vi "TimeSampleDlgg.vi"() -> (2 "定时采样信息":T1)   [LabVIEW 2014, in "Sample.lvlib"]
uses:
  Sample.lvlib
  DataBase/DataBase.lvlib
panel:
  in  "备注":string
  out "电压范围":string
  in  "取消按钮":bool
  in  "确定按钮":bool
  in  "电源频率（Hz）":string="1"
  in  "电源电压":string
  in  "分钟":u16(ring) items=["0", "01", "02", "03", "04", "05", "06", "07", "08", "09", "10", "11", "12", "13", "14", "15", "16", "17", "18", "19", "20", "21", "22", "23", "24", "25", "26", "27", "28", "29", "30", "31", "32", "33", "34", "35", "36", "37", "38", "39", "40", "41", "42", "43", "44", "45", "46", "47", "48", "49", "50", "51", "52", "53", "54", "55", "56", "57", "58", "59"]
  in  "时":u16(ring) items=["1", "2", "3", "4", "5", "6", "7", "8", "9", "10", "11", "12", "13", "14", "15", "16", "17", "18", "19", "20", "21", "22", "23", "24"]
  in  "检测区域":string(combo)
  in  "是否启动":string(combo)="是"
  in  "检测位置":string(combo)="上层膜检测"
  in  "OK":bool
  # "检测时间"
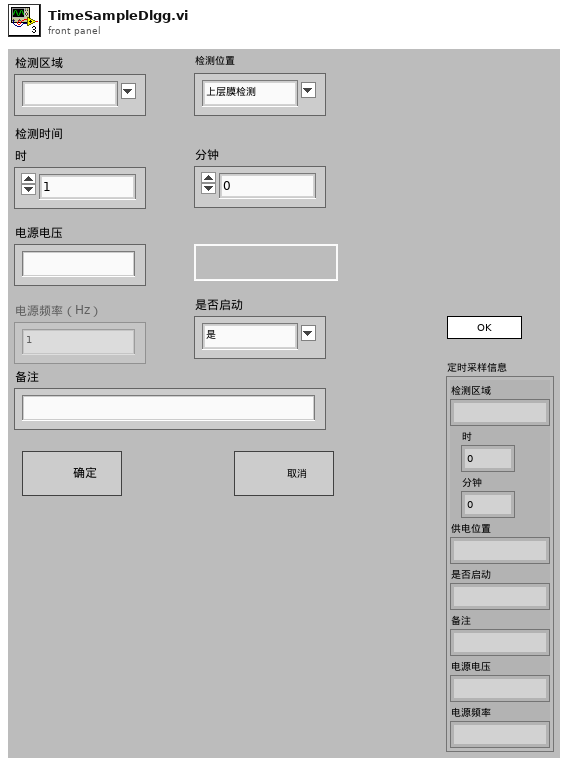
[diagram p1: front panel]
types:
  T1 = cluster{"检测区域":string, "时":u16, "分钟":u16, "供电位置":string, "是否启动":string, "备注":string, "电源电压":string, "电源频率":string}
  T2 = enum32{"invalid app kind", "Development System", "Run Time System", "Student Edition", "Embedded LabVIEW", "Evaluation", "Custom"}
  T3 = enum32{"Invalid", "Standard", "Closed", "Hidden", "Minimized", "Maximized"}
  T4 = cluster{"Core":cluster{"Current VI Reference":refnum<vi>, "Close Panel on Exit?":bool}, "Your Boolean data":bool, "Your string data":string, "AreaName":string, "SampleAreaName":string[], "定时采样信息":cluster{"检测区域":string, "时":u16, "分钟":u16, "供电位置":string, "是否启动":string, "备注":string, "电源电压":string, "电源频率":string}, "电源倍数":string, "最大电压值":i32}
  T5 = cluster{"Current VI Reference":refnum<vi>, "Close Panel on Exit?":bool}
  T6 = cluster{string, "检测区域":string, "供电位置":string, string, string, "是否启动":string, "电源电压":string, "电源频率":string, "备注":string}
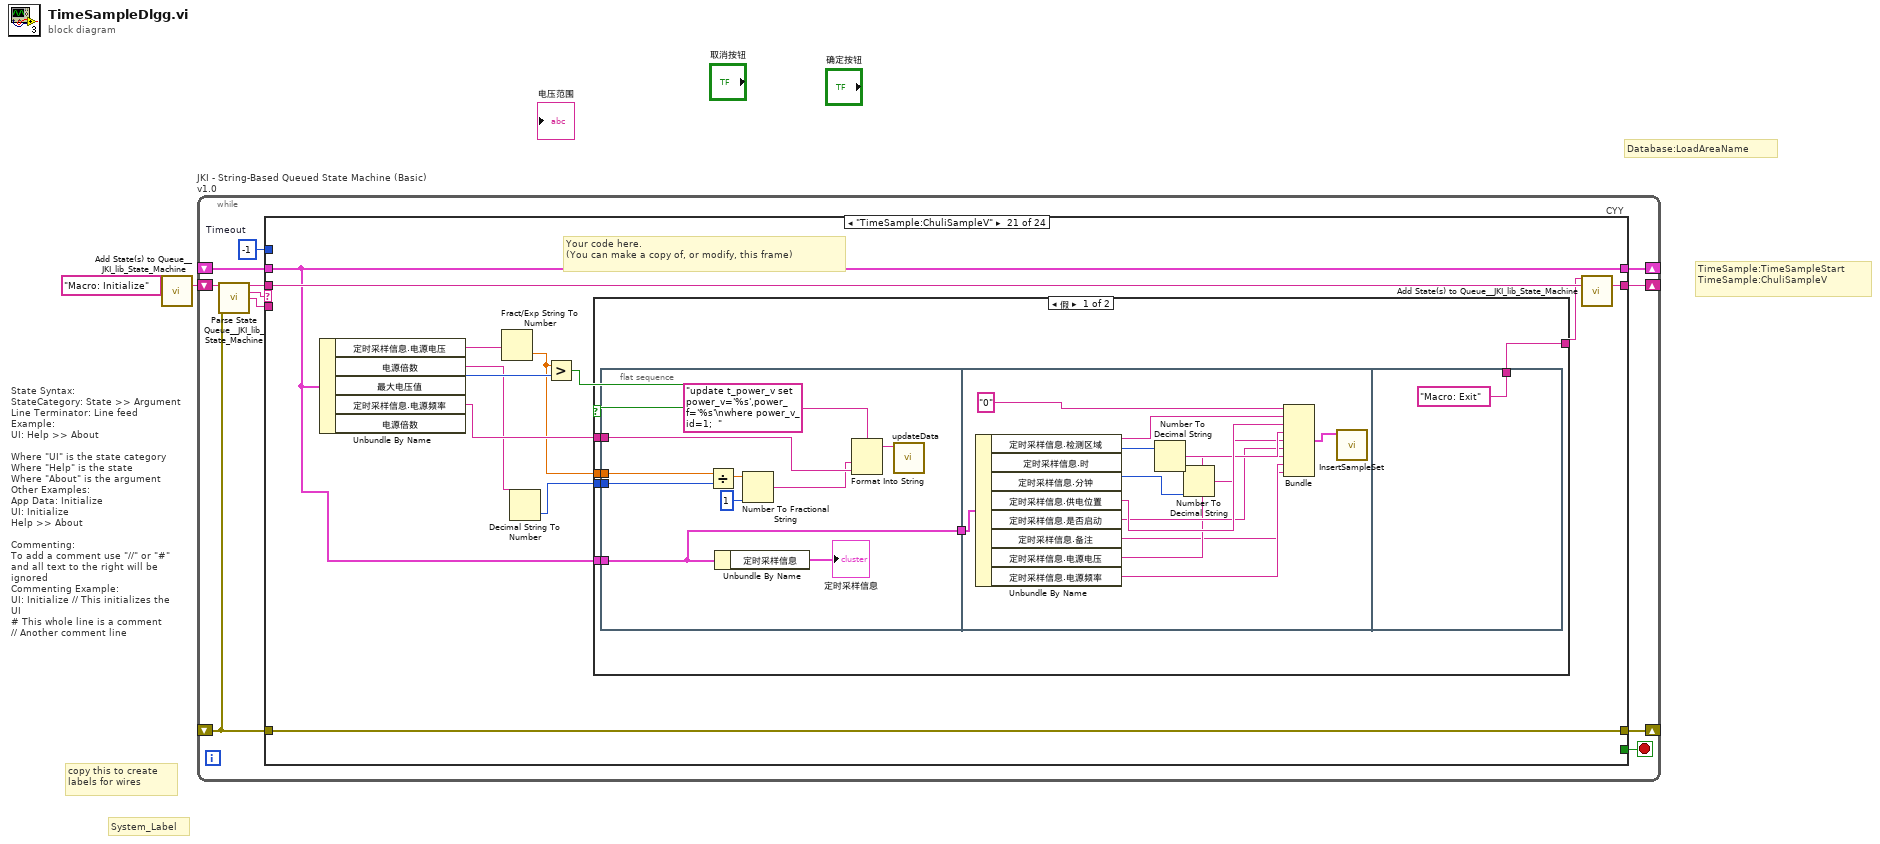
[diagram p0: block diagram]
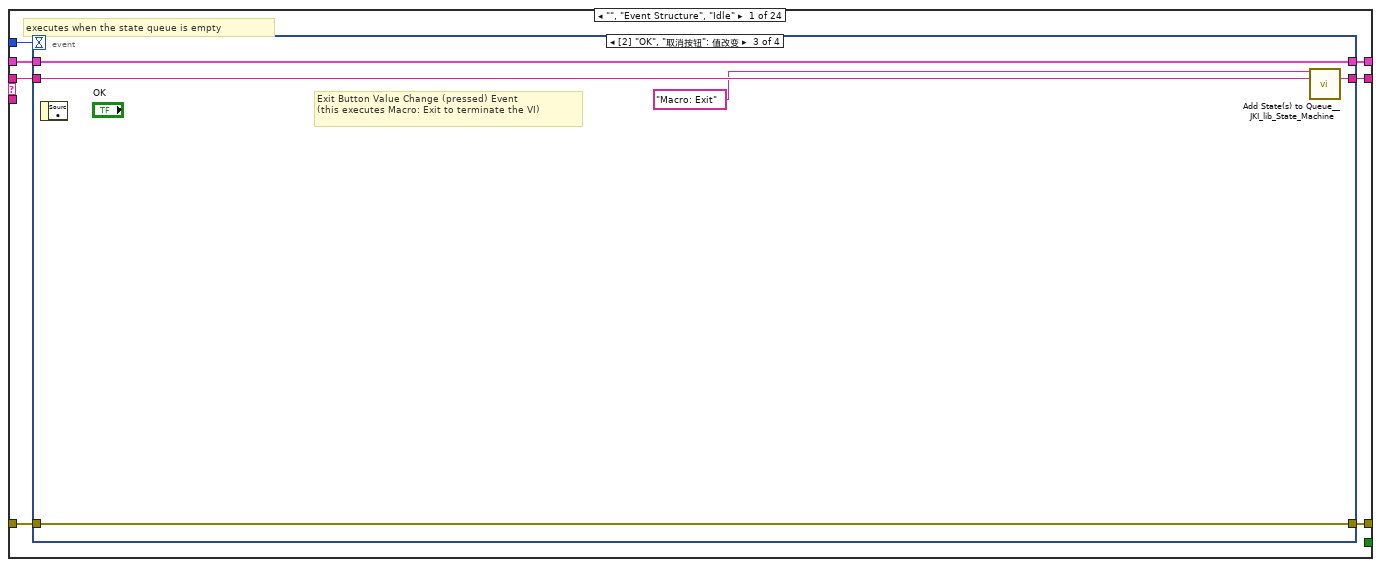
[diagram p2: hidden frame]
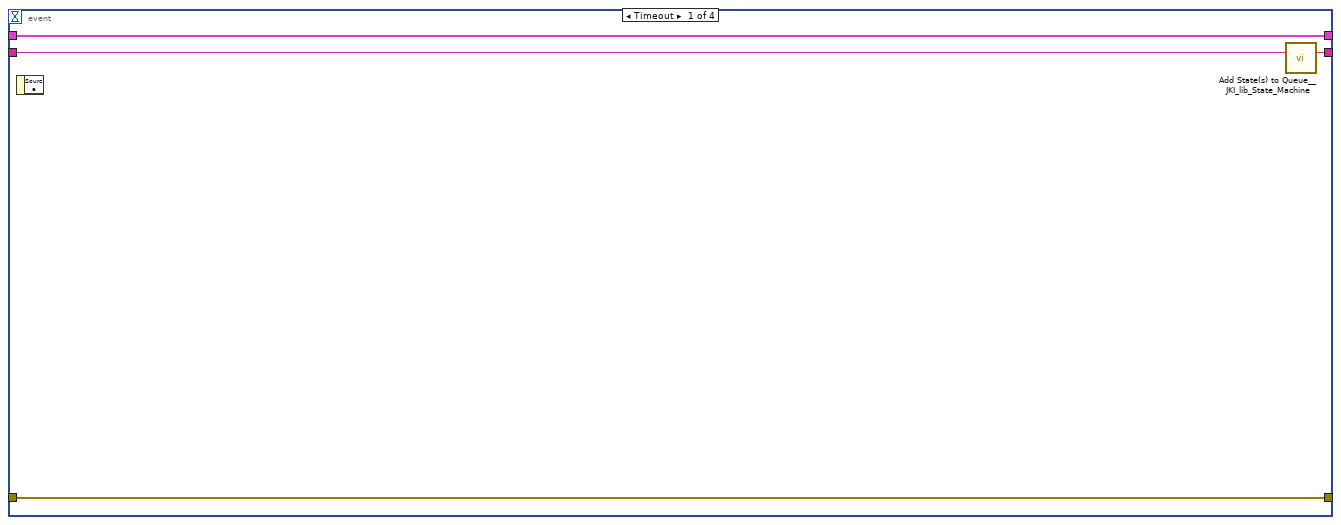
[diagram p3: hidden frame]
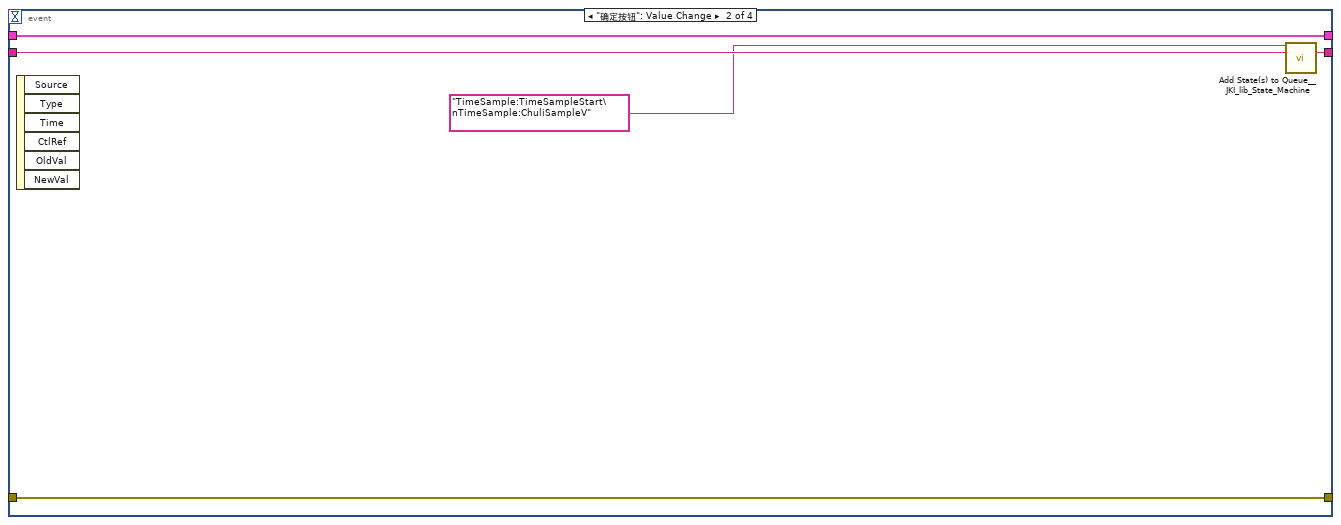
[diagram p4: hidden frame]
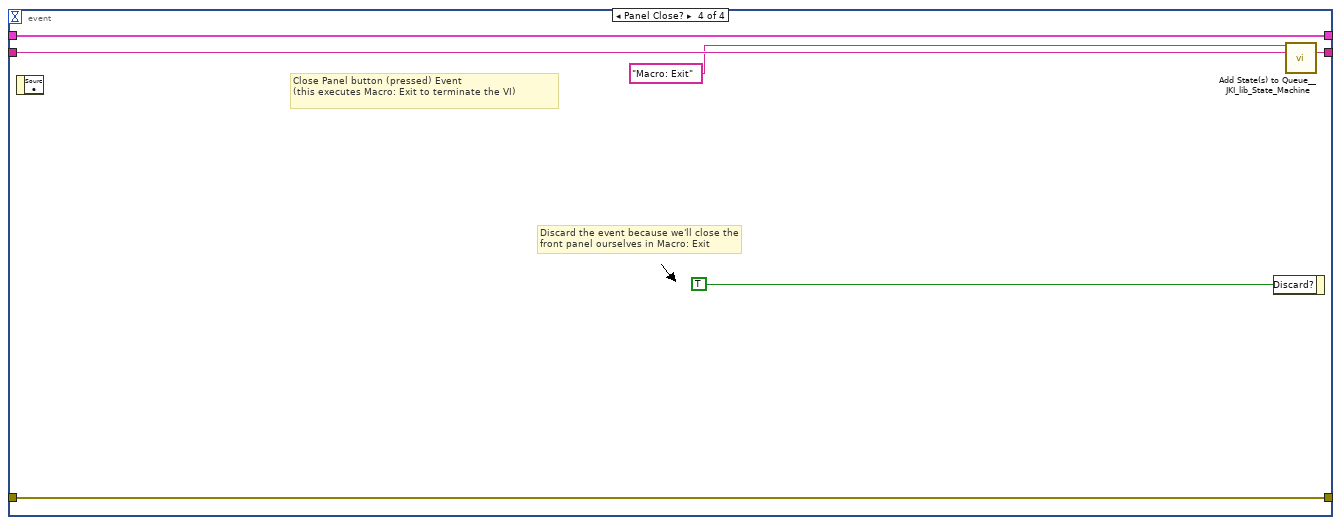
[diagram p5: hidden frame]
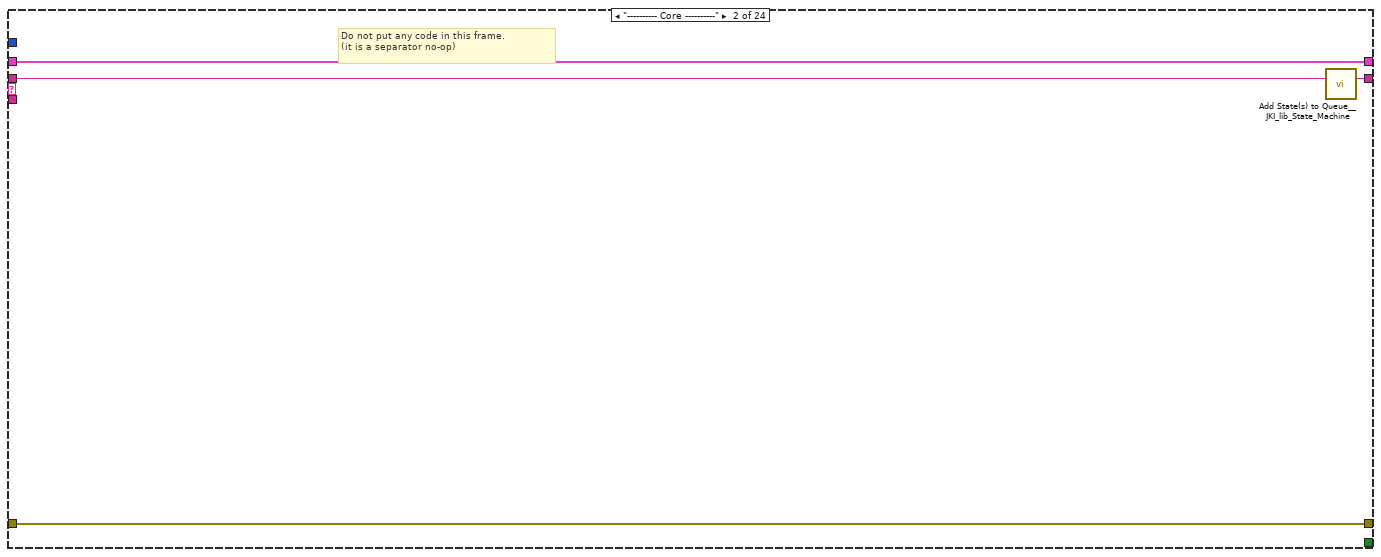
[diagram p6: hidden frame]
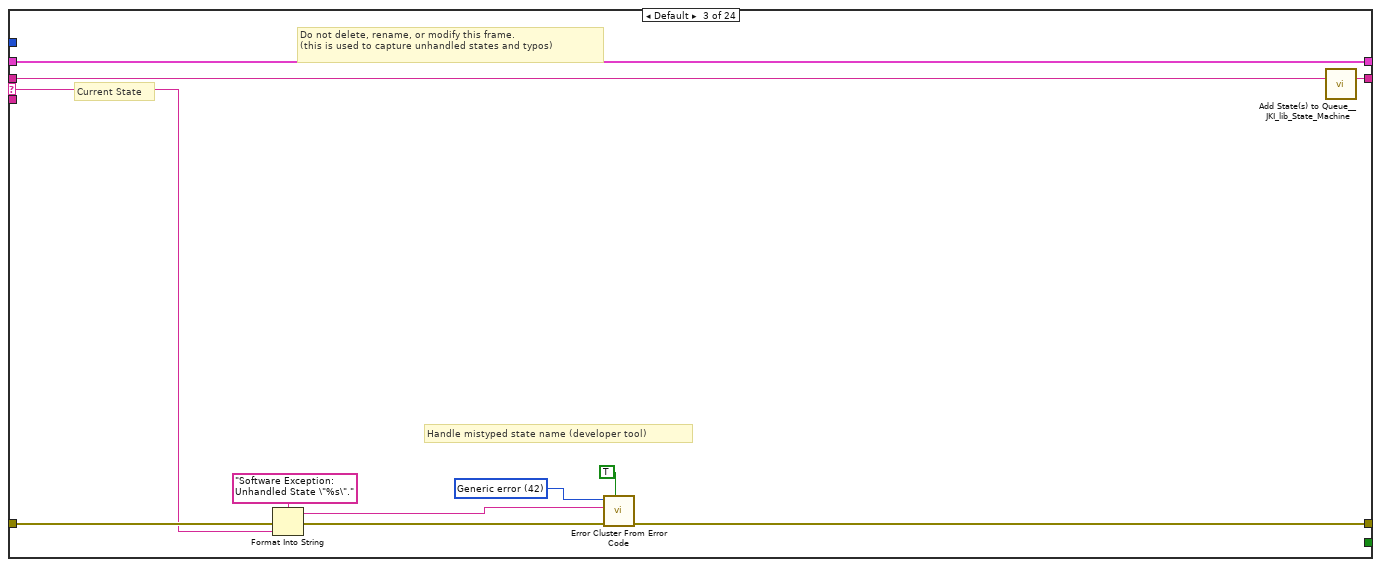
[diagram p7: hidden frame]
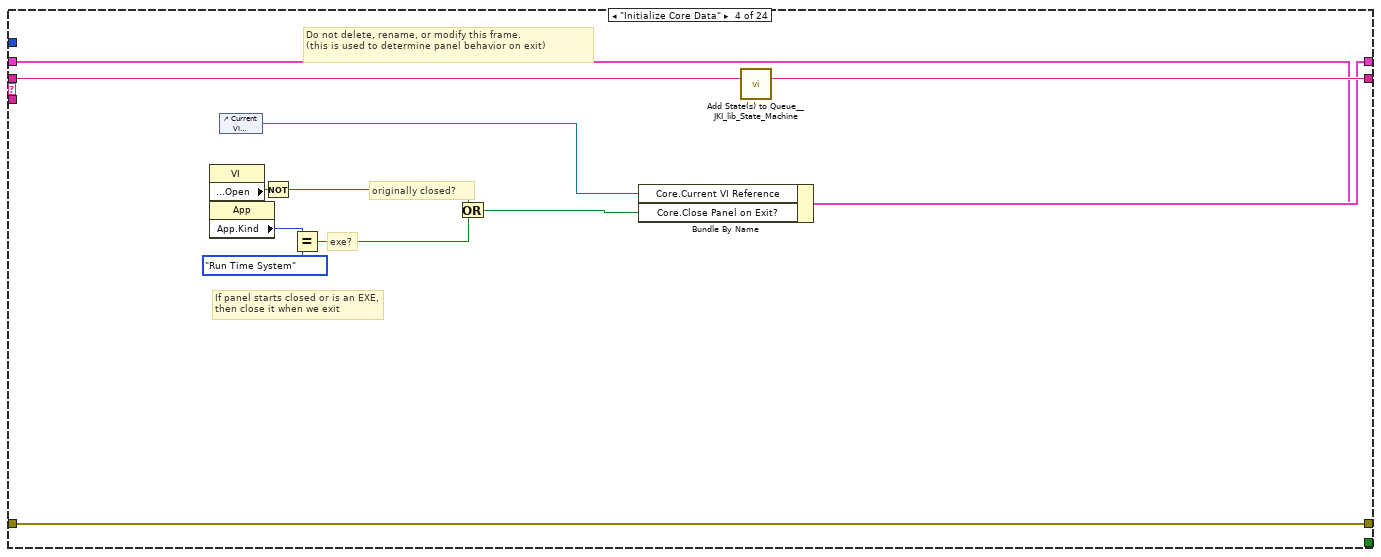
[diagram p8: hidden frame]
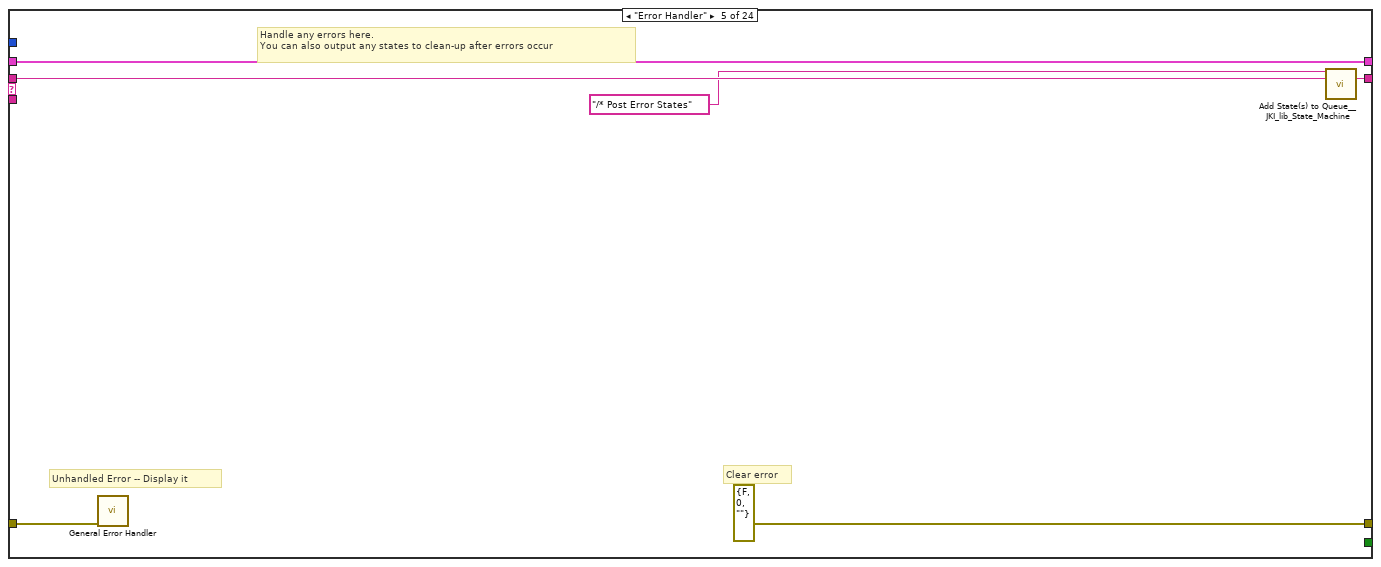
[diagram p9: hidden frame]
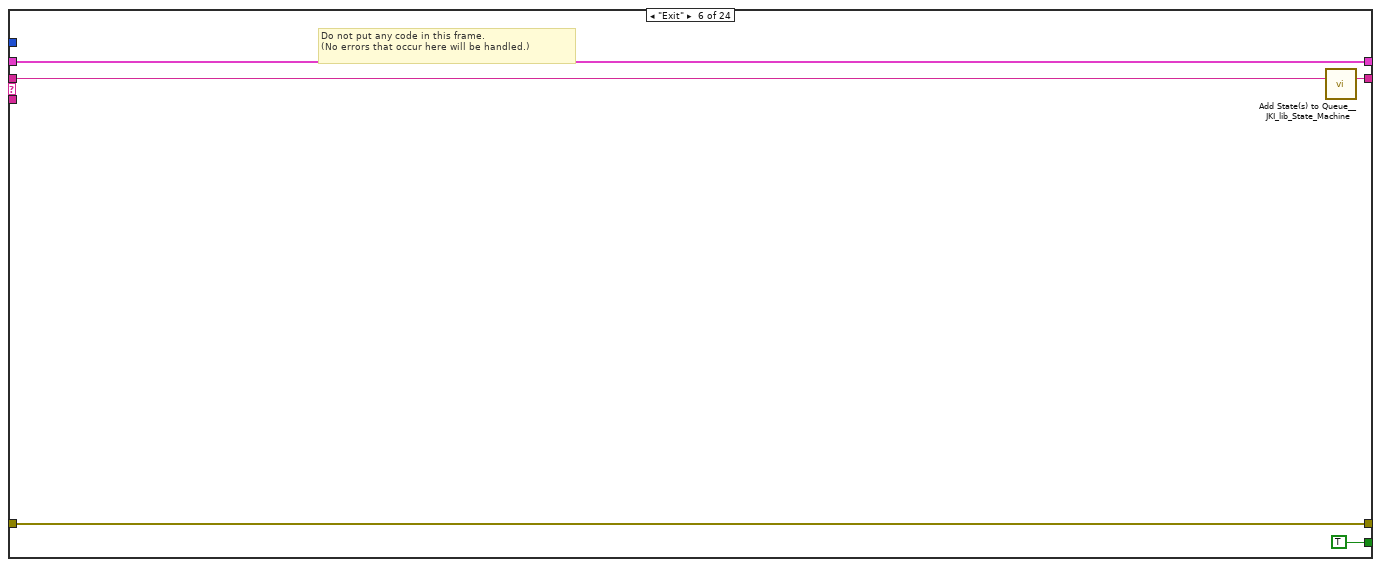
[diagram p10: hidden frame]
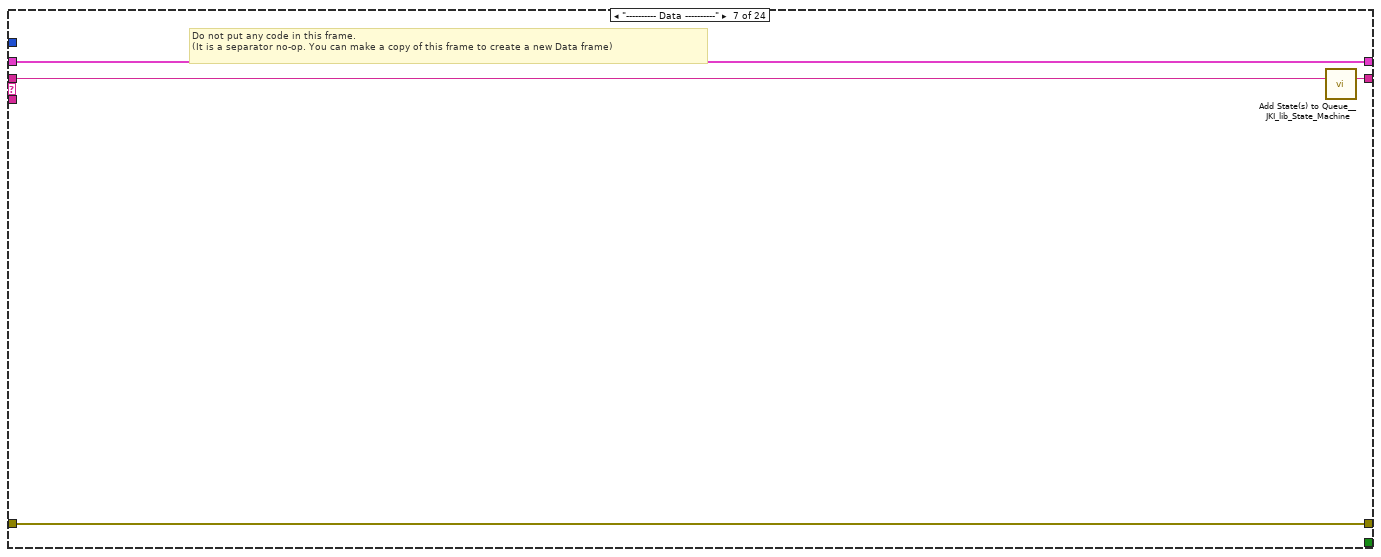
[diagram p11: hidden frame]
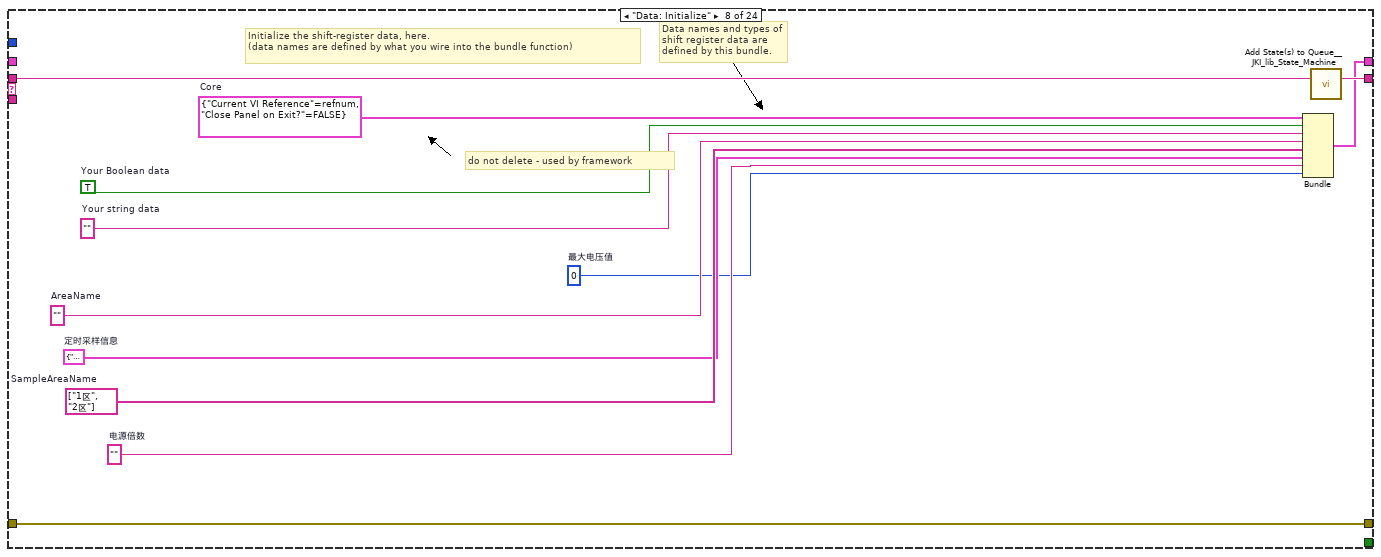
[diagram p12: hidden frame]
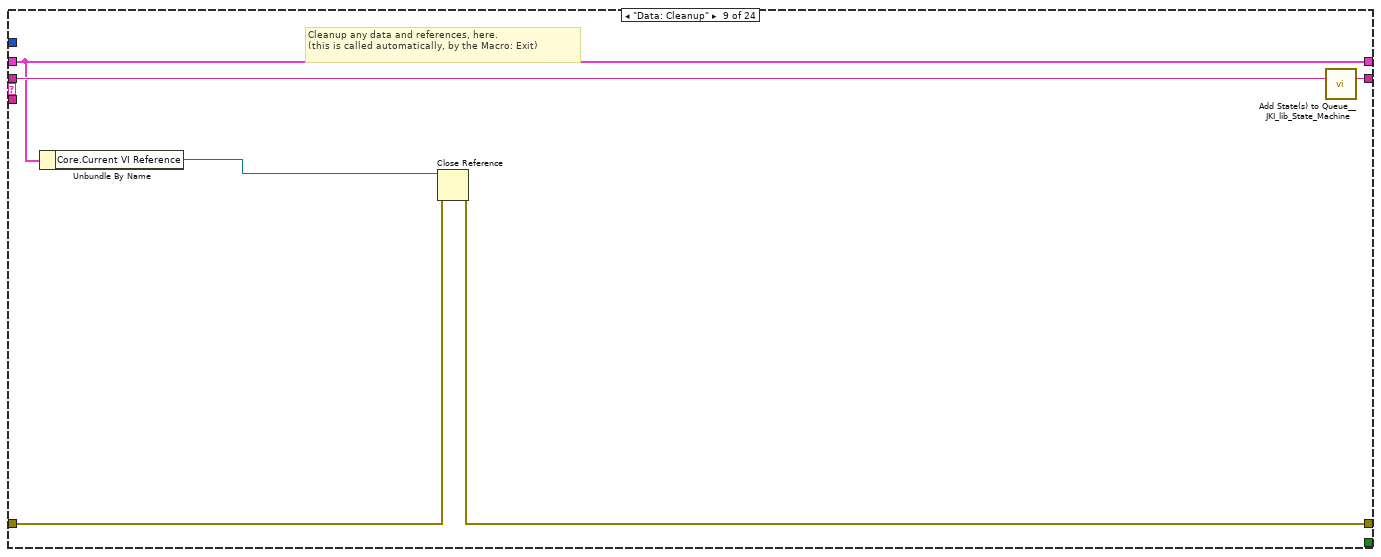
[diagram p13: hidden frame]
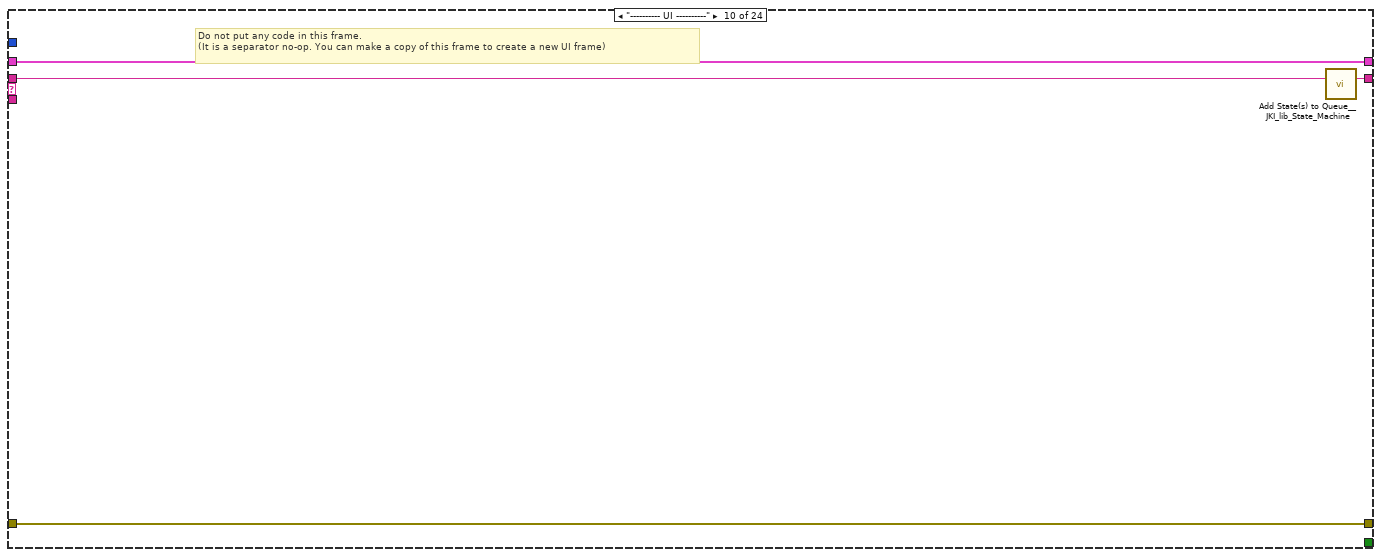
[diagram p14: hidden frame]
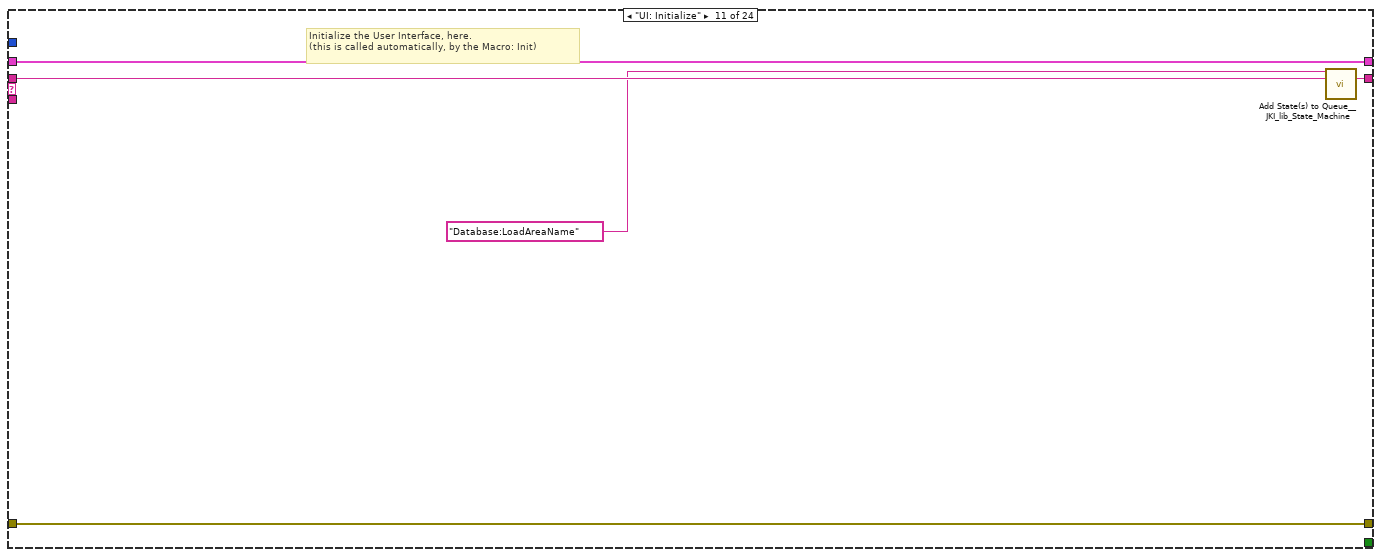
[diagram p15: hidden frame]
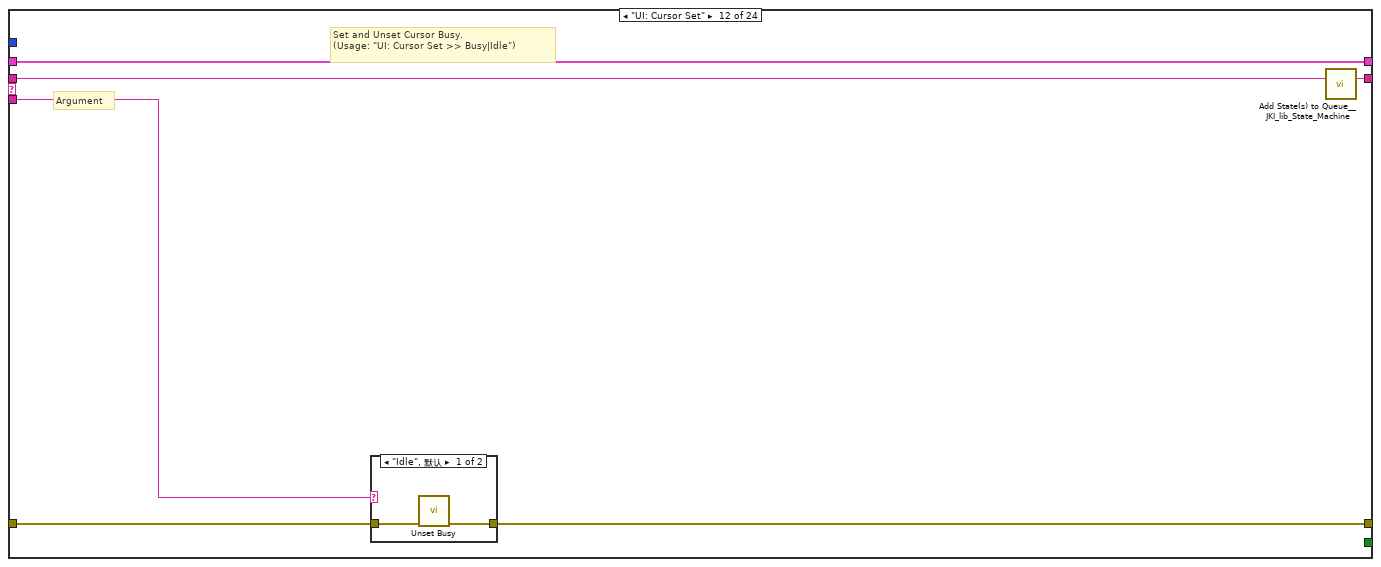
[diagram p16: hidden frame]
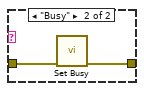
[diagram p17: hidden frame]
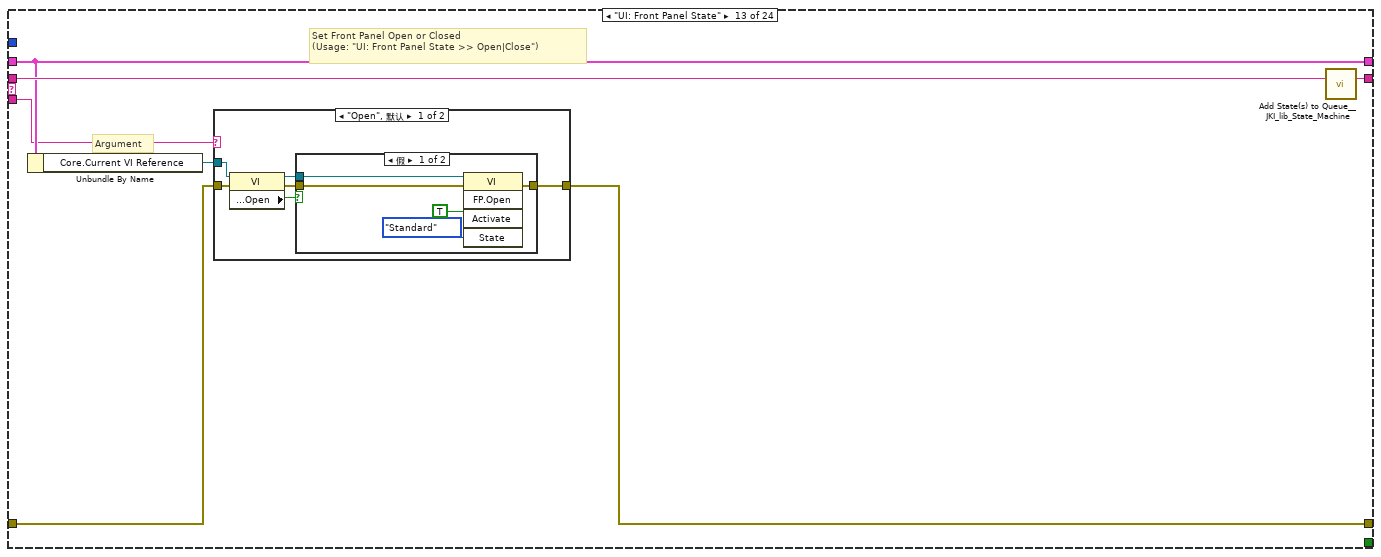
[diagram p18: hidden frame]
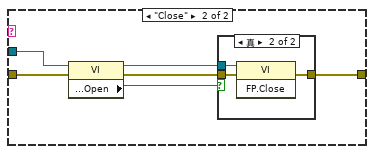
[diagram p20: hidden frame]
diagram:
  # "TimeSample:TimeSampleStart\nTimeSample:ChuliSampleV"
  # "Database:LoadAreaName"
  # "State Syntax:\nStateCategory: State >> Argument\nLine Terminator: Line feed\nExample:\nUI: Help >> About\n\nWhere \"UI\" is the state category\nWhere \"Help\" is the state\nWhere \"About\" is the argument\nOther Examples:\nApp Data: Initialize\nUI: Initialize\nHelp >> About\n\nCommenting:\nTo add a comment use \"//\" or \"#\" and all text to the right will be ignored\nCommenting Example:\nUI: Initialize // This initializes the UI\n# This whole line is a comment\n// Another comment line"
  # "copy this to create labels for wires"
  # "System_Label"
  n1 = call <vilib>:"Add State(s) to Queue__JKI_lib_State_Machine.vi"("State(s) in (\"\")"="Macro: Initialize") -> ("States Out"=w2:string)  [unwired: 14 in]
  n2 = while "JKI - String-Based Queued State Machine (Basic) v1.0" {
    shift-right: [w6] -> _
    shift-left: _ -> [w5]
    shift-right: [w9] -> _
    shift-left: _ -> [w3]
    shift-right: [w8] -> _
    shift-left: w2 -> [w10]
    stop <- w7 stop-if-true
    w4 = -1  # Timeout
    # "CYY"
    n3 = call <vilib>:"Parse State Queue__JKI_lib_State_Machine.vi"("State Queue"=w10, "Error In (no error)"=w3) -> ("Remaining States"=w12:string, "Current State"=w13:string, "Arguments"=w11:string)  [unwired: 11 in]
    n4 = case shown="\"TimeSample:ChuliSampleV\"" w13 {
      selector: w13 -> [_ _ w45 _ _ _ _ _ _ _ _ _ _ _ _ _ _ _ _ _ _ _ _ _]
      tunnel: w12 -> [w20 w44 w49 w67 w73 w78 w82 w94 w100 w104 w109 w115 w126 w152 w157 w167 w171 w175 w179 w183 w195 w241 w245 w255]
      tunnel: w11 -> [_ _ _ _ _ _ _ _ _ _ _ w110 w120 _ _ _ _ _ _ _ _ _ _ _]
      tunnel: w5 -> [w18 w41 w47 w58 w70 w76 w79 _ w95 w101 w107 w113 w122 w149 w154 w164 w168 w172 w176 w180 w184 w229 w242 w252]
      tunnel: [w17 w42 w51 w64 errorcluster {"status"=FALSE, "code"=0, "source"=""} ("error out") w75 w80 w91 w96 w102 w106 w111 w123 w150 w155 w165 w169 w173 w177 w181 w193 w239 w243 w253] -> w9
      tunnel: w3 -> [w16 w42 w50 w64 w69 w75 w80 w91 w97 w102 w106 w112 w124 w150 w155 w165 w169 w173 w177 w181 w193 w239 w243 w253]
      tunnel: [w19 w43 w48 w66 w72 w77 w81 w93 w99 w103 w108 w114 w125 w151 w156 w166 w170 w174 w178 w182 w194 w240 w244 w254] -> w8
      tunnel: [_ _ _ _ _ TRUE _ _ _ _ _ _ _ _ _ _ _ _ _ _ _ _ _ _] -> w7
      tunnel: [w15 w41 w47 w65 w70 w76 w79 w92 w95 w101 w107 w113 w122 w149 w154 w164 w168 w172 w176 w180 w184 w238 w242 w251] -> w6
      tunnel: w4 -> [w14 _ _ _ _ _ _ _ _ _ _ _ _ _ _ _ _ _ _ _ _ _ _ _]
      frame "", "Event Structure", "Idle" {
        # "executes when the state queue is empty"
        n5 = event shown="[2] \"OK\", \"取消按钮\": 值改变" {
          selector: _ -> [_ _ _ _]
          dyn-events: _ -> [_ _ _ _]
          timeout: w14 -> [_ _ _ _]
          tunnel: w20 -> [w24 w29 w34 w40]
          tunnel: [w23 w28 w33 w39] -> w19
          tunnel: w18 -> [w21 w26 w31 w37]
          tunnel: [w22 w27 w32 w38] -> w17
          tunnel: w16 -> [w22 w27 w32 w38]
          tunnel: [w21 w26 w31 w37] -> w15
          event Timeout {
            n6 = event-data() -> ()  [unwired: 1 in, 1 out]
            n7 = call <vilib>:"Add State(s) to Queue__JKI_lib_State_Machine.vi"("State(s) in (\"\")"=w24) -> ("States Out"=w23:string)  [unwired: 14 in]
          }
          event "确定按钮": Value Change {
            n8 = event-data() -> ()  [unwired: 1 in, 6 out]
            n9 = call <vilib>:"Add State(s) to Queue__JKI_lib_State_Machine.vi"("State(s) in Front (\"\")"="TimeSample:TimeSampleStart\nTimeSample:ChuliSampleV", "State(s) in (\"\")"=w29) -> ("States Out"=w28:string)  [unwired: 13 in]
          }
          event "OK", "取消按钮": Value Change {
            # "Exit Button Value Change (pressed) Event\n(this executes Macro: Exit to terminate the VI)"
            n10 = event-data() -> ()  [unwired: 1 in, 1 out]
            n11 = call <vilib>:"Add State(s) to Queue__JKI_lib_State_Machine.vi"("State(s) in Front (\"\")"="Macro: Exit", "State(s) in (\"\")"=w34) -> ("States Out"=w33:string)  [unwired: 13 in]
          }
          event Panel Close? {
            # "Discard the event because we'll close the front panel ourselves in Macro: Exit"
            # "Close Panel button (pressed) Event\n(this executes Macro: Exit to terminate the VI)"
            n12 = event-data() -> ()  [unwired: 1 in, 1 out]
            n13 = event-data("Discard?"=TRUE) -> ()  [unwired: 1 in, 1 out]
            n14 = call <vilib>:"Add State(s) to Queue__JKI_lib_State_Machine.vi"("State(s) in Front (\"\")"="Macro: Exit", "State(s) in (\"\")"=w40) -> ("States Out"=w39:string)  [unwired: 13 in]
          }
        }
      }
      frame "---------- Core ----------" {
        # "Do not put any code in this frame.\n(it is a separator no-op)"
        n15 = call <vilib>:"Add State(s) to Queue__JKI_lib_State_Machine.vi"("State(s) in (\"\")"=w44) -> ("States Out"=w43:string)  [unwired: 14 in]
      }
      frame Default {
        w54 = 42 items=["No error", "Argument error", "Memory is full", "Out of zone", "End of file", "File already open", "Generic file I/O error", "File not found", "File permission error", "Disk is full", "Duplicate path", "Too many files open", "System feature not enabled", "Resource file not found", "Cannot add resource", "Resource not found", "Image not found", "Image memory error", "Pen does not exist", "Config type invalid", "Config token not found", "Config parse error", "Config memory error", "Bad external code format", "Bad external code offset", "External code not present", "Null window", "Destroy window error", "Null menu", "Print aborted", "Bad print record", "Print driver error", "Windows error during printing", "Memory error during printing", "Print dialog error", "Generic print error", "Invalid device refnum", "Device not found", "Device parameter error", "Device unit error", "Cannot open device", "Device call aborted", "Generic error", "Cancelled by user", "Object ID too low", "Object ID too high", "Object not in heap", "Unknown heap", "Unknown object (invalid DefProc)", "Unknown object (DefProc not in table)", "Message out of range", "Invalid (null) method", "Unknown message", "Manager call not supported", "Bad address", "Network operation in progress", "Network operation timed out", "Connection is busy", "Network attribute not supported", "Network error", "Address in use", "System out of memory", "Connection aborted", "Connection refused", "Not connected", "Already connected", "Connection closed", "Initialization error (interapplication manager)", "Bad occurrence", "Wait on unbound occurrence handler", "Occurrence queue overflow", "Datalog type conflict", "Unused", "Unrecognized type (interapplication manager)", "Memory corrupt", "Failed to make temporary DLL", "Old CIN version", "Drag socket not found", "Failed to load drop-object", "Failed to register OLE object", "Failed to release OLE object", "Format specifier type mismatch", "Unknown format specifier", "Too few format specifiers", "Too many format specifiers", "Scan failed", "Newer CIN version", "Error converting to variant", "Runtime menu error", "Password tampered", "Variant attribute not found", "Incompatible variant data type", "Event data is not available", "Event Store is not present", "Occurrence is not found", "Event Queue is not created", "Event info is not available", "Refnum passed is NULL", "Error retrieving Class GUID", "Error retrieving CoClass GUID", "Error retrieving TypeLib GUID.", "Bad built application magic bytes.", "Specific driver is different from the specific driver associated with the Logical Name.", "There is no session opened to the class driver.", "Max Error", "MAX - Error with config objects", "MAX - Error loading configuration", "MAX - Group not supported"]
        # "Current State"
        # "Do not delete, rename, or modify this frame.\n(this is used to capture unhandled states and typos)"
        # "Handle mistyped state name (developer tool)"
        n16 = Format Into String(format string="Software Exception: Unhandled State \"%s\"." ("message"), error in=w50, w45) -> (resulting string=w53:string, error out=w52:errorcluster)  [unwired: 1 in]
        n17 = call <vilib>:"Error Cluster From Error Code.vi"("show call chain? (False)"=TRUE, "error in (no error)"=w52, "error message (\"\")"=w53, "error code (0)"=w54) -> ("error out"=w51:errorcluster)  [unwired: 5 in]
        n18 = call <vilib>:"Add State(s) to Queue__JKI_lib_State_Machine.vi"("State(s) in (\"\")"=w49) -> ("States Out"=w48:string)  [unwired: 14 in]
      }
      frame "Initialize Core Data" {
        # "Do not delete, rename, or modify this frame.\n(this is used to determine panel behavior on exit)"
        # "originally closed?"
        # "exe?"
        # "If panel starts closed or is an EXE, then close it when we exit"
        n19 = property class="VI"() -> ("Front Panel.Open"=w63:bool)  [unwired: 2 in, 2 out]
        n20 = property class="App"() -> ("App.Kind"=w62:T2)  [unwired: 2 in, 2 out]
        n21 = control-ref of="Current VI Reference"() -> (w56:refnum<vi>)
        n22 = Not(x=w63) -> (.not. x?=w60:bool)
        n23 = Equal?(x=w62, y=T2."Run Time System" ("Application:Kind")) -> (x = y?=w59:bool)
        n24 = Or(x=w60, y=w59) -> (x .or. y?=w57:bool)
        n25 = Bundle By Name(cluster=w58, "Core.Current VI Reference"=w56, "Core.Close Panel on Exit?"=w57) -> (w65:T4)
        n26 = call <vilib>:"Add State(s) to Queue__JKI_lib_State_Machine.vi"("State(s) in (\"\")"=w67) -> ("States Out"=w66:string)  [unwired: 14 in]
      }
      frame "Error Handler" {
        # "Unhandled Error -- Display it"
        # "Handle any errors here.\nYou can also output any states to clean-up after errors occur"
        # "Clear error"
        n27 = call <vilib>:"General Error Handler.vi"("error in (no error)"=w69) -> ()  [unwired: 10 in, 5 out]
        n28 = call <vilib>:"Add State(s) to Queue__JKI_lib_State_Machine.vi"("State(s) in Front (\"\")"="/* Post Error States", "State(s) in (\"\")"=w73) -> ("States Out"=w72:string)  [unwired: 13 in]
      }
      frame "Exit" {
        # "Do not put any code in this frame.\n(No errors that occur here will be handled.)"
        n29 = call <vilib>:"Add State(s) to Queue__JKI_lib_State_Machine.vi"("State(s) in (\"\")"=w78) -> ("States Out"=w77:string)  [unwired: 14 in]
      }
      frame "---------- Data ----------" {
        # "Do not put any code in this frame.\n(It is a separator no-op. You can make a copy of this frame to create a new Data frame)"
        n30 = call <vilib>:"Add State(s) to Queue__JKI_lib_State_Machine.vi"("State(s) in (\"\")"=w82) -> ("States Out"=w81:string)  [unwired: 14 in]
      }
      frame "Data: Initialize" {
        w83 = 0  # 最大电压值
        w84 = ""  # 电源倍数
        w85 = T1 {"检测区域"="", "时"=0, "分钟"=0, "供电位置"="", "是否启动"="", "备注"="", "电源电压"="", "电源频率"=""}  # 定时采样信息
        w86 = string[] ["1区", "2区"]  # SampleAreaName
        w87 = ""  # AreaName
        w88 = T5 {"Current VI Reference"=refnum, "Close Panel on Exit?"=FALSE}  # Core
        w90 = TRUE  # Your Boolean data
        w89 = ""  # Your string data
        # "do not delete - used by framework"
        # "Data names and types of shift register data are defined by this bundle."
        # "Initialize the shift-register data, here.\n(data names are defined by what you wire into the bundle function)"
        n31 = Bundle("Core"=w88, "Your Boolean data"=w90, "Your string data"=w89, "AreaName"=w87, "SampleAreaName"=w86, "定时采样信息"=w85, "电源倍数"=w84, "最大电压值"=w83) -> (w92:T4)  [unwired: 1 in]
        n32 = call <vilib>:"Add State(s) to Queue__JKI_lib_State_Machine.vi"("State(s) in (\"\")"=w94) -> ("States Out"=w93:string)  [unwired: 14 in]
      }
      frame "Data: Cleanup" {
        # "Cleanup any data and references, here.\n(this is called automatically, by the Macro: Exit)"
        n33 = Unbundle By Name(w95) -> ("Core.Current VI Reference"=w98:refnum<vi>)
        n34 = Close Reference(reference=w98, error in (no error)=w97) -> (error out=w96:errorcluster)
        n35 = call <vilib>:"Add State(s) to Queue__JKI_lib_State_Machine.vi"("State(s) in (\"\")"=w100) -> ("States Out"=w99:string)  [unwired: 14 in]
      }
      frame "---------- UI ----------" {
        # "Do not put any code in this frame.\n(It is a separator no-op. You can make a copy of this frame to create a new UI frame)"
        n36 = call <vilib>:"Add State(s) to Queue__JKI_lib_State_Machine.vi"("State(s) in (\"\")"=w104) -> ("States Out"=w103:string)  [unwired: 14 in]
      }
      frame "UI: Initialize" {
        # "Initialize the User Interface, here.\n(this is called automatically, by the Macro: Init)"
        n37 = call <vilib>:"Add State(s) to Queue__JKI_lib_State_Machine.vi"("State(s) in Front (\"\")"="Database:LoadAreaName", "State(s) in (\"\")"=w109) -> ("States Out"=w108:string)  [unwired: 13 in]
      }
      frame "UI: Cursor Set" {
        # "Argument"
        # "Set and Unset Cursor Busy.\n(Usage: \"UI: Cursor Set >> Busy|Idle\")"
        n38 = case shown="\"Idle\", 默认" w110 {
          tunnel: w112 -> [w117 w119]
          tunnel: [w116 w118] -> w111
          frame "Idle", Default {
            n39 = call <vilib>:"Unset Busy.vi"("error in (no error)"=w117) -> ("error out"=w116:errorcluster)  [unwired: 10 in]
          }
          frame "Busy" {
            n40 = call <vilib>:"Set Busy.vi"("error in (no error)"=w119) -> ("error out"=w118:errorcluster)  [unwired: 9 in, 1 out]
          }
        }
        n41 = call <vilib>:"Add State(s) to Queue__JKI_lib_State_Machine.vi"("State(s) in (\"\")"=w115) -> ("States Out"=w114:string)  [unwired: 14 in]
      }
      frame "UI: Front Panel State" {
        # "Argument"
        # "Set Front Panel Open or Closed\n(Usage: \"UI: Front Panel State >> Open|Close\")"
        n42 = Unbundle By Name(w122) -> ("Core.Current VI Reference"=w121:refnum<vi>)
        n43 = case shown="\"Open\", 默认" w120 {
          tunnel: w124 -> [w130 w143]
          tunnel: [w132 w144] -> w123
          tunnel: w121 -> [w131 w141]
          frame "Open", Default {
            n44 = property class="VI"(reference=w131, error in=w130) -> (reference out=w128:refnum<vi>, error out=w129:errorcluster, "Front Panel.Open"=w127:bool)
            n45 = case shown="假" w127 {
              tunnel: [w135 w138] -> w132
              tunnel: w129 -> [w134 w138]
              tunnel: w128 -> [w133 _]
              frame False {
                n46 = invoke class="VI" method="FP.Open"(reference=w133, error in=w134, "Activate"=TRUE, "State"=T3."Standard") -> (error out=w135:errorcluster)  [unwired: 1 in, 4 out]
              }
              frame True {
              }
            }
          }
          frame "Close" {
            n47 = property class="VI"(reference=w141, error in=w143) -> (reference out=w140:refnum<vi>, error out=w142:errorcluster, "Front Panel.Open"=w139:bool)
            n48 = case shown="真" w139 {
              tunnel: [w145 w148] -> w144
              tunnel: w142 -> [w145 w147]
              tunnel: w140 -> [_ w146]
              frame False {
              }
              frame True {
                n49 = invoke class="VI" method="FP.Close"(reference=w146, error in=w147) -> (error out=w148:errorcluster)  [unwired: 1 in, 2 out]
              }
            }
          }
        }
        n50 = call <vilib>:"Add State(s) to Queue__JKI_lib_State_Machine.vi"("State(s) in (\"\")"=w126) -> ("States Out"=w125:string)  [unwired: 14 in]
      }
      frame "---------- Macro ----------" {
        # "Do not put any code in this frame.\n(It is a separator no-op. You can make a copy of this frame to create a new Macro frame)"
        n51 = call <vilib>:"Add State(s) to Queue__JKI_lib_State_Machine.vi"("State(s) in (\"\")"=w152) -> ("States Out"=w151:string)  [unwired: 14 in]
      }
      frame "Macro: Initialize" {
        w153 = "Data: Initialize\nInitialize Core Data\nUI: Initialize\nUI: Front Panel State >> Open"  # Data: Initialize Initialize Core Data UI: Initialize UI: Front Panel State >> Open
        # "Initialization Macro\n(This is called once, when the VI starts)"
        n52 = call <vilib>:"Add State(s) to Queue__JKI_lib_State_Machine.vi"("State(s) in Front (\"\")"=w153, "State(s) in (\"\")"=w157) -> ("States Out"=w156:string)  [unwired: 13 in]
      }
      frame "Macro: Exit" {
        # "Exit Macro\n(This is called once, when the VI exits)"
        n53 = Unbundle By Name(w164) -> ("Core.Close Panel on Exit?"=w163:bool)
        n54 = Select(t="UI: Front Panel State >> Close", s=w163, f="") -> (s? t:f=w160:string)
        n55 = call <vilib>:"Add State(s) to Queue__JKI_lib_State_Machine.vi"("State(s) in (\"\")"=w160, "State(s) at Back (\"\")"="Data: Cleanup\nExit") -> ("States Out"=w158:string)  [unwired: 13 in]
        n56 = call <vilib>:"Add State(s) to Queue__JKI_lib_State_Machine.vi"("State(s) in Front (\"\")"=w158, "State(s) in (\"\")"=w167) -> ("States Out"=w166:string)  [unwired: 13 in]
      }
      frame "---------- New Category ----------" {
        # "Template Separator\n(You can make a copy of, or modify, this frame)"
        n57 = call <vilib>:"Add State(s) to Queue__JKI_lib_State_Machine.vi"("State(s) in (\"\")"=w171) -> ("States Out"=w170:string)  [unwired: 14 in]
      }
      frame "New Category: 1" {
        # "Your code here.\n(You can make a copy of, or modify, this frame)"
        n58 = call <vilib>:"Add State(s) to Queue__JKI_lib_State_Machine.vi"("State(s) in (\"\")"=w175) -> ("States Out"=w174:string)  [unwired: 14 in]
      }
      frame "New Category: 2" {
        # "Your code here.\n(You can make a copy of, or modify, this frame)"
        n59 = call <vilib>:"Add State(s) to Queue__JKI_lib_State_Machine.vi"("State(s) in (\"\")"=w179) -> ("States Out"=w178:string)  [unwired: 14 in]
      }
      frame "---------TimeSample--------" {
        # "Your code here.\n(You can make a copy of, or modify, this frame)"
        n60 = call <vilib>:"Add State(s) to Queue__JKI_lib_State_Machine.vi"("State(s) in (\"\")"=w183) -> ("States Out"=w182:string)  [unwired: 14 in]
      }
      frame "TimeSample:ChuliSampleV" {
        # "Your code here.\n(You can make a copy of, or modify, this frame)"
        n61 = Unbundle By Name(w184) -> ("定时采样信息.电源电压"=w192:string, "电源倍数"=w186:string, "最大电压值"=w191:i32, "定时采样信息.电源频率"=w188:string)  [unwired: 1 out]
        n62 = Fract/Exp String To Number(string=w192) -> (number=w187:dbl)  [unwired: 3 in, 1 out]
        n63 = Decimal String To Number(string=w186) -> (number=w185:i32)  [unwired: 2 in, 1 out]
        n64 = Greater?(x=w187, y=w191) -> (0:w190:bool)
        n65 = case shown="假" w190 {
          tunnel: [w197 ""] -> w189
          tunnel: w188 -> [w201 _]
          tunnel: w187 -> [w200 _]
          tunnel: w185 -> [w199 _]
          tunnel: w184 -> [w198 _]
          frame False {
            n66 = flat-sequence {
              tunnel: w201 -> [w209]
              tunnel: w200 -> [w206]
              tunnel: w199 -> [w205]
              tunnel: w198 -> [w202]
              tunnel: [w202] -> w196
              tunnel: w196 -> [w223]
              tunnel: ["Macro: Exit"] -> w197
              frame #0 {
                n67 = Divide(x=w206, y=w205) -> (x/y=w208:dbl)
                n68 = Unbundle By Name(w202) -> ("定时采样信息"=→"定时采样信息":T1)
                n69 = Number To Fractional String(number=w208, precision (6)=i16 1 ("精度(6)")) -> (F-format string=w204:string)  [unwired: 2 in]
                n70 = Format Into String(format string="update t_power_v set power_v='%s',power_f='%s'\nwhere power_v_id=1;  ", w204, w209) -> (resulting string=w211:string)  [unwired: 2 in, 1 out]
                n71 = call "updateData.vi"("SQL query"=w211) -> ()  [unwired: 10 in, 1 out]
              }
              frame #1 {
                n72 = Unbundle By Name(w223) -> ("定时采样信息.检测区域"=w222:string, "定时采样信息.时"=w221:u16, "定时采样信息.分钟"=w220:u16, "定时采样信息.供电位置"=w219:string, "定时采样信息.是否启动"=w216:string, "定时采样信息.备注"=w213:string, "定时采样信息.电源电压"=w215:string, "定时采样信息.电源频率"=w214:string)
                n73 = Number To Decimal String(number=w221) -> (decimal integer string=w218:string)  [unwired: 1 in]
                n74 = Number To Decimal String(number=w220) -> (decimal integer string=w217:string)  [unwired: 1 in]
                n75 = Bundle("0", "检测区域"=w222, "供电位置"=w219, w218, w217, "是否启动"=w216, "电源电压"=w215, "电源频率"=w214, "备注"=w213) -> (w212:T6)  [unwired: 1 in]
                n76 = call "InsertSampleSet.vi"("SampleSet"=w212) -> ()  [unwired: 10 in, 1 out]
              }
              frame #2 {
              }
            }
          }
          frame True {
            n77 = One Button Dialog(message="电压超过范围，请从新输入") -> ()  [unwired: 1 in, 1 out]
          }
        }
        n78 = call <vilib>:"Add State(s) to Queue__JKI_lib_State_Machine.vi"("State(s) in Front (\"\")"=w189, "State(s) in (\"\")"=w195) -> ("States Out"=w194:string)  [unwired: 13 in]
      }
      frame "TimeSample:TimeSampleStart" {
        # "Your code here.\n(You can make a copy of, or modify, this frame)"
        n79 = Increment(x="时") -> (x+1=w235:u16)
        n80 = Bundle By Name(cluster=w229, "定时采样信息.检测区域"="检测区域", "定时采样信息.时"=w235, "定时采样信息.分钟"="分钟", "定时采样信息.供电位置"="检测位置", "定时采样信息.是否启动"="是否启动", "定时采样信息.备注"="备注", "定时采样信息.电源电压"="电源电压", "定时采样信息.电源频率"="电源频率（Hz）") -> (w238:T4)
        n81 = call <vilib>:"Add State(s) to Queue__JKI_lib_State_Machine.vi"("State(s) in (\"\")"=w241) -> ("States Out"=w240:string)  [unwired: 14 in]
      }
      frame "----------Database---------" {
        # "Your code here.\n(You can make a copy of, or modify, this frame)"
        n82 = call <vilib>:"Add State(s) to Queue__JKI_lib_State_Machine.vi"("State(s) in (\"\")"=w245) -> ("States Out"=w244:string)  [unwired: 14 in]
      }
      frame "Database:LoadAreaName" {
        # "Your code here.\n(You can make a copy of, or modify, this frame)"
        n83 = control-ref of="检测区域"() -> (w250:refnum<vi>)
        n84 = call "GetVandBeishu.vi"() -> ("电压倍数"=w247:string)  [unwired: 9 in, 2 out]
        n85 = call "GetDBAreaName.vi"("ComboBox输入"=w250) -> ("所有记录"=w249:string[])  [unwired: 9 in, 1 out]
        n86 = call "ZhuanVbeishu.vi"("电压倍数"=w247) -> ("电压范围"=w246:string, "最大电压值"=w248:i32)  [unwired: 9 in]
        n87 = Bundle By Name(cluster=w252, "SampleAreaName"=w249, "电源倍数"=w247, "最大电压值"=w248) -> (w251:T4)
        n88 = property on="电压范围" class="Str"("Text.Text"=w246) -> ()  [unwired: 2 in, 2 out]
        n89 = call <vilib>:"Add State(s) to Queue__JKI_lib_State_Machine.vi"("State(s) in (\"\")"=w255) -> ("States Out"=w254:string)  [unwired: 14 in]
      }
    }
  }
